vi "Get API.vi"(8 "error in (no error)":errorcluster, 11 "TCPMessaging in":refnum<class "TCPMessaging.lvclass">) -> (0 "error out":errorcluster, 2 "TCP Service API":refnum<class "TCPMessageAPI.lvclass">, 3 "TCPMessaging out":refnum<class "TCPMessaging.lvclass">)   [LabVIEW 2020, in "Vecto.lvlib" / "TCPMessaging.lvclass"]
uses:
  TCPMessaging.lvclass
  TCPMessageService/TCPMessageAPI.lvclass
  TCPMessaging.lvclass/TCPMessaging.ctl
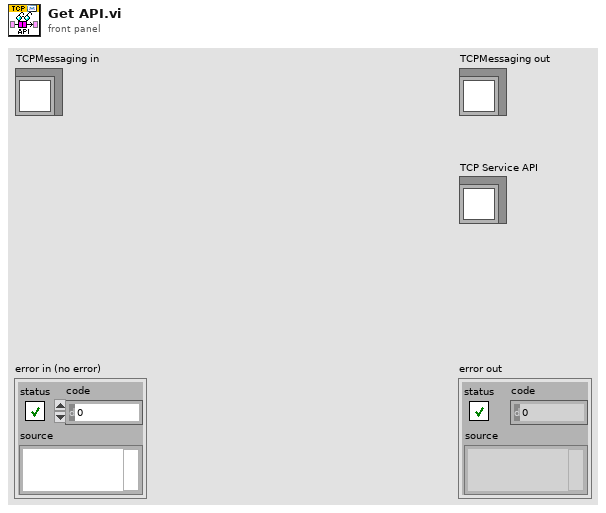
[diagram p1: front panel]
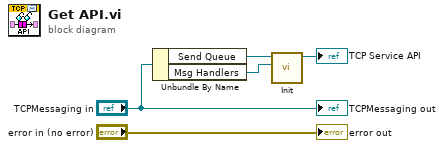
[diagram p0: block diagram]
diagram:
  n1 = Unbundle By Name("TCPMessaging in") -> ("Send Queue"=w3:refnum<queue>, "Msg Handlers"=w1:refnum<queue>)
  n2 = call "Init.vi"("Msg Handlers"=w1, "Send Queue"=w3) -> ("TCPMessageService out"=→"TCP Service API":refnum<class "TCPMessageAPI.lvclass">)  [unwired: 8 in, 1 out]
  "error out" <- "error in (no error)"
  "TCPMessaging out" <- "TCPMessaging in"
